vi "Disabled Property(Main Controls)_Measure.vi"(8 "error in (no error)":errorcluster, 11 "MWWL Verification in":refnum<class "MWWL Verification.lvclass">) -> (0 "error out":errorcluster, 3 "MWWL Verification out":refnum<class "MWWL Verification.lvclass">)   [LabVIEW 2018, in "MWWL Verification.lvlib" / "MWWL Verification.lvclass"]
uses:
  MWWL Verification.lvclass
  MWWL Verification.lvclass/MWWL Verification.ctl
types:
  T1 = enum8{"Enabled", "Disabled", "Disabled and Grayed Out"}
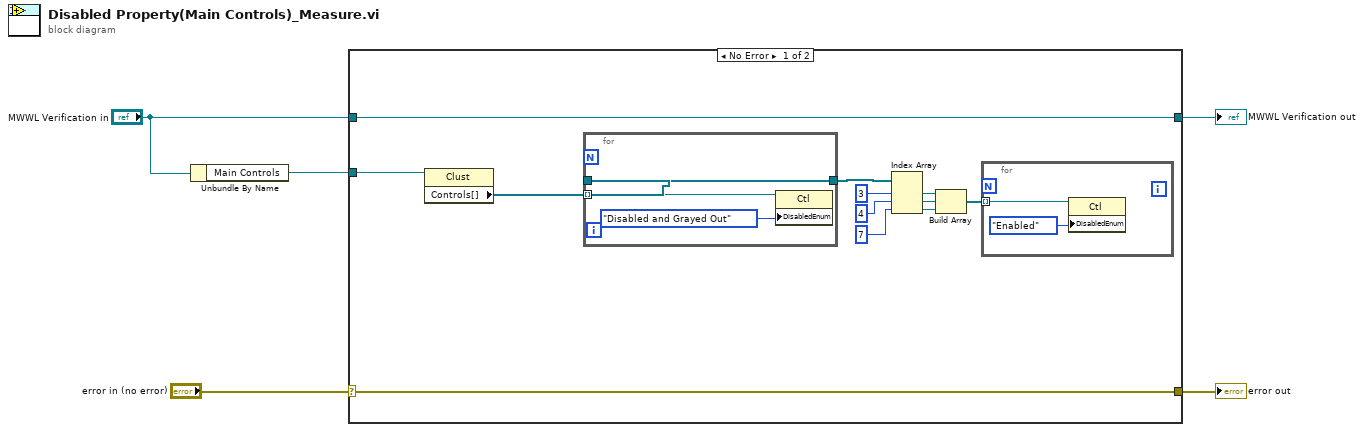
[diagram p0: block diagram]
diagram:
  n1 = Unbundle By Name("MWWL Verification in") -> ("Main Controls"=w1:refnum<vi>)
  n2 = case shown="No Error" "error in (no error)" {
    selector: "error in (no error)" -> [w16 w24]
    tunnel: [w16 w24] -> w4
    tunnel: [w17 w23] -> w3
    tunnel: "MWWL Verification in" -> [w17 w23]
    tunnel: w1 -> [w15 _]
    frame No Error {
      n3 = property class="Clust"(reference=w15) -> ("Controls[]"=w13:refnum<vi>[])  [unwired: 1 in, 2 out]
      n4 = for {
        tunnel: w13 -> [w21] mode=indexing
        tunnel: [w20] -> w12
        tunnel: w13 -> [w20]
        n5 = property class="Ctl"(reference=w21, "DisabledEnum"=T1."Disabled and Grayed Out" ("Disabled")) -> ()  [unwired: 1 in, 2 out]
      }
      n6 = Index Array(array=w12, index #1=3 ("index"), index #2=4 ("index"), index #3=7 ("index")) -> (element #1=w9:refnum<vi>, element #2=w8:refnum<vi>, element #3=w7:refnum<vi>)
      n7 = Build Array(w9, w8, w7) -> (w6:refnum<vi>[])
      n8 = for {
        tunnel: w6 -> [w18] mode=indexing
        n9 = property class="Ctl"(reference=w18, "DisabledEnum"=T1."Enabled" ("Disabled")) -> ()  [unwired: 1 in, 2 out]
      }
    }
    frame Error {
    }
  }
  "error out" <- w4
  "MWWL Verification out" <- w3
